vi "Crossover (Pixel).vi"(1 "Father":u8[](array[numeric]) format="0x%02x", 2 "Mother":u8[](array[numeric]) format="0x%02x") -> (0 "Child":u8[](array[numeric]) format="0x%02x")   [LabVIEW 2013]
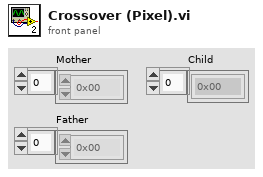
[diagram p1: front panel]
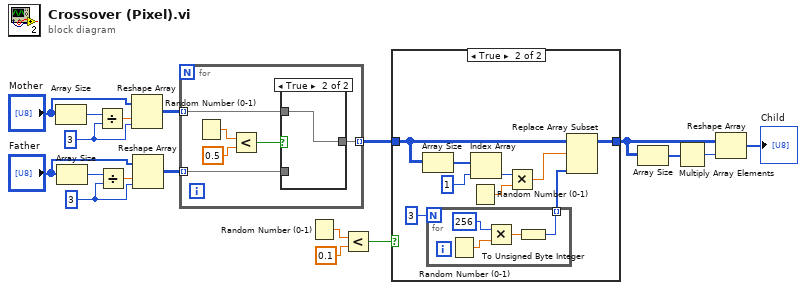
[diagram p0: block diagram]
diagram:
  w7 = 3
  w11 = 3
  n1 = Array Size(array="Mother") -> (size(s)=w12:i32)
  n2 = Array Size(array="Father") -> (size(s)=w8:i32)
  n3 = Divide(x=w12, y=w11) -> (x/y=w13:dbl)
  n4 = Divide(x=w8, y=w7) -> (x/y=w9:dbl)
  n5 = Reshape Array("Mother", w13, w11) -> (w14:u8[][])
  n6 = Reshape Array("Father", w9, w7) -> (w6:u8[][])
  n7 = for {
    tunnel: w14 -> [w20] mode=indexing
    tunnel: w6 -> [w21] mode=indexing
    tunnel: [w19] -> w18 mode=indexing
    n8 = Random Number (0-1)() -> (number: 0 to 1=w23:dbl)
    n9 = Less?(x=w23, y=0.5) -> (x < y?=w22:bool)
    n10 = case shown="True" w22 {
      tunnel: w21 -> [w25 _]
      tunnel: w20 -> [_ w26]
      tunnel: [w25 w26] -> w19
      frame False {
      }
      frame True {
      }
    }
  }
  n11 = Random Number (0-1)() -> (number: 0 to 1=w17:dbl)
  n12 = Less?(x=w17, y=0.1) -> (x < y?=w15:bool)
  n13 = case shown="True" w15 {
    tunnel: w18 -> [w27 w35]
    tunnel: [w27 w36] -> w2
    frame False {
    }
    frame True {
      n14 = Array Size(array=w35) -> (size(s)=w31:i32[])
      n15 = for {
        N: 3 -> [_]
        tunnel: [w38] -> w33 mode=indexing
        n16 = Random Number (0-1)() -> (number: 0 to 1=w40:dbl)
        n17 = Multiply(x=256, y=w40) -> (x*y=w37:dbl)
        n18 = To Unsigned Byte Integer(number=w37) -> (unsigned 8bit integer=w38:u8)
      }
      n19 = Random Number (0-1)() -> (number: 0 to 1=w34:dbl)
      n20 = Index Array(array=w31, index=1) -> (element=w30:i32)
      n21 = Multiply(x=w30, y=w34) -> (x*y=w28:dbl)
      n22 = Replace Array Subset(array=w35, new element=w33, index (row)=w28) -> (w36:u8[][])  [unwired: 1 in]
    }
  }
  n23 = Array Size(array=w2) -> (size(s)=w4:i32[])
  n24 = Multiply Array Elements(1:w4) -> (0:w3:i32)
  n25 = Reshape Array(w2, w3) -> (→"Child":u8[])
